vi "PWM to CAN.vi"(4 "manual/wysylanie":bool, 8 "cluster manipulator 2":T4, 11 "Cluster":T2={"MANIPULATOR ID 3 "=3, "0 bajt"=1, "serwa i pompa"={"4"=TRUE, "1 "=TRUE, "3"=TRUE, "2"=TRUE, "lewy"=TRUE, "serwo 3"=TRUE, "serwo 4 "=TRUE, "przekaznik"=TRUE}}) -> (1 "array of cans":T3[](array[typedef]) {"type" items=["CAN Data", "CAN Remote"]; "identifier" format="%.0x"}, 2 "druga ramka manipulator":T3 {"type" items=["CAN Data", "CAN Remote"]; "identifier" format="%.0x"}, 3 "Pierwsza ramka manipulator":T3 {"type" items=["CAN Data", "CAN Remote"]; "identifier" format="%.0x"})   [LabVIEW 2015]
uses:
  RT/CANFrameControl.ctl
  klapki.ctl
panel:
  out "unsigned 8bit integer":u8
  out "0, 1":i16[](array[numeric])
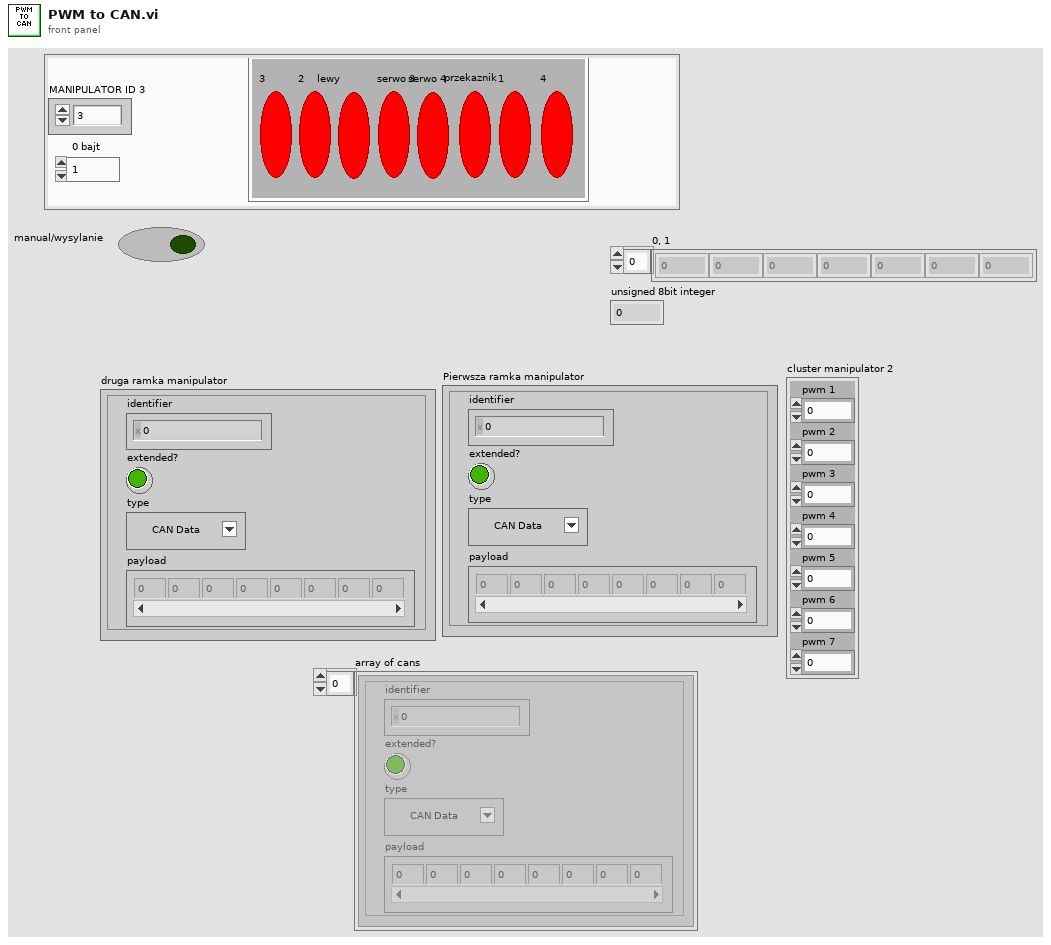
[diagram p1: front panel]
types:
  T1 = typedef "klapki.ctl" = cluster{"4":bool, "1 ":bool, "3":bool, "2":bool, "lewy":bool, "serwo 3":bool, "serwo 4 ":bool, "przekaznik":bool}
  T2 = cluster{"MANIPULATOR ID 3 ":u32, "0 bajt":u8, "serwa i pompa":T1}
  T3 = typedef "CANFrameControl.ctl" = cluster{"identifier":u32, "extended?":bool, "type":u8, "payload":u8[]}
  T4 = cluster{"pwm 1":dbl, "pwm 2":dbl, "pwm 3":dbl, "pwm 4":dbl, "pwm 5":dbl, "pwm 6":dbl, "pwm 7":dbl}
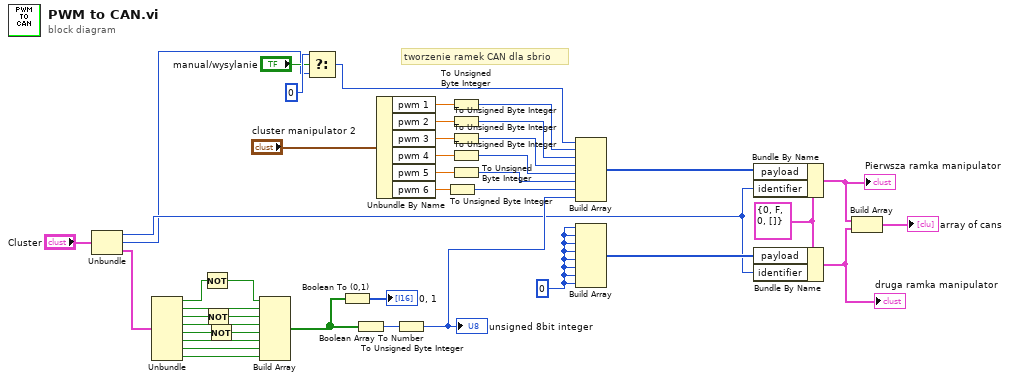
[diagram p0: block diagram]
diagram:
  w9 = u8 0
  w36 = T3 {"identifier"=0, "extended?"=FALSE, "type"=0, "payload"=[]} ("CAN frame 2")
  # "tworzenie ramek CAN dla sbrio"
  n1 = Unbundle("Cluster") -> ("MANIPULATOR ID 3"=w7:u32, "0 bajt"=w6:u8, "serwa i pompa"=w5:T1)
  n2 = Unbundle(w5) -> ("4"=w3:bool, "1"=w16:bool, "3"=w2:bool, "2"=w23:bool, "lewy"=w14:bool, "serwo 3"=w19:bool, "serwo 4"=w15:bool, "przekaznik"=w18:bool)
  n3 = Not(x=w3) -> (.not. x?=w4:bool)
  n4 = Not(x=w2) -> (.not. x?=w1:bool)
  n5 = Not(x=w14) -> (.not. x?=w13:bool)
  n6 = Build Array(w4, w16, w1, w23, w13, w19, w15, w18) -> (w17:bool[])
  n7 = Select(t=u8 0, s="manual/wysylanie", f=w6) -> (s? t:f=w10:u8)
  n8 = Boolean To (0,1)(Boolean=w17) -> (0, 1=→"0, 1":i16[])
  n9 = Boolean Array To Number(Boolean array=w17) -> (number=w22:u32)
  n10 = Unbundle By Name("cluster manipulator 2") -> ("pwm 1"=w41:dbl, "pwm 2"=w40:dbl, "pwm 3"=w39:dbl, "pwm 4"=w38:dbl, "pwm 5"=w37:dbl, "pwm 6"=w31:dbl)
  n11 = To Unsigned Byte Integer(number=w22) -> (unsigned 8bit integer=w20:u8)
  "unsigned 8bit integer" <- w20
  n12 = To Unsigned Byte Integer(number=w31) -> (unsigned 8bit integer=w25:u8)
  n13 = To Unsigned Byte Integer(number=w41) -> (unsigned 8bit integer=w30:u8)
  n14 = To Unsigned Byte Integer(number=w40) -> (unsigned 8bit integer=w29:u8)
  n15 = To Unsigned Byte Integer(number=w39) -> (unsigned 8bit integer=w28:u8)
  n16 = To Unsigned Byte Integer(number=w38) -> (unsigned 8bit integer=w27:u8)
  n17 = To Unsigned Byte Integer(number=w37) -> (unsigned 8bit integer=w26:u8)
  n18 = Build Array(w10, w30, w29, w28, w27, w26, w25, w20) -> (w24:u8[])
  n19 = Build Array(w9, w9, w9, w9, w9, w9, w9, w9) -> (w35:u8[])
  n20 = Bundle By Name(cluster=w36, "payload"=w24, "identifier"=w7) -> (w33:T3)
  "Pierwsza ramka manipulator" <- w33
  n21 = Bundle By Name(cluster=w36, "payload"=w35, "identifier"=w7) -> (w32:T3)
  "druga ramka manipulator" <- w32
  n22 = Build Array(w33, w32) -> (→"array of cans":T3[])
